vi "ConfigureArmTrigger.vi"(8 "Error In":errorcluster, 10 "Arm Configuration":T1={"Source"=enum."Hold", "Count"=1, "Infinite?"=FALSE} {"Count" min=1 max=99999 step=1}, 11 "Keithley 7001 In":refnum<visa-resource-name>) -> (0 "Error Out":errorcluster, 3 "Keithley 7001 Out":refnum<visa-resource-name>)   [LabVIEW 2012]
uses:
  TriggerArmConfiguration.ctl
  driver/Public/Controls/ArmSource.ctl
  driver/Keithley-7001.lvlib
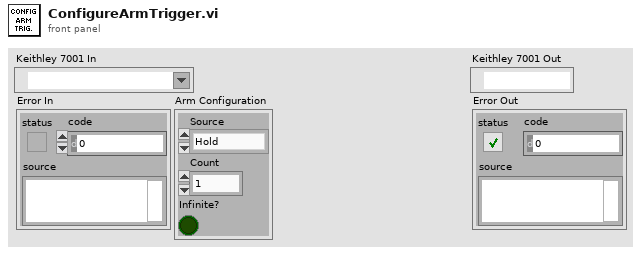
[diagram p1: front panel]
types:
  T1 = typedef "TriggerArmConfiguration.ctl" = cluster{"Source":T2, "Count":u32, "Infinite?":bool}
  T2 = typedef "Keithley-7001.lvlib/ArmSource.ctl" = enum16{"Hold", "Immediate", "Manual", "Bus", "TLink", "External"}
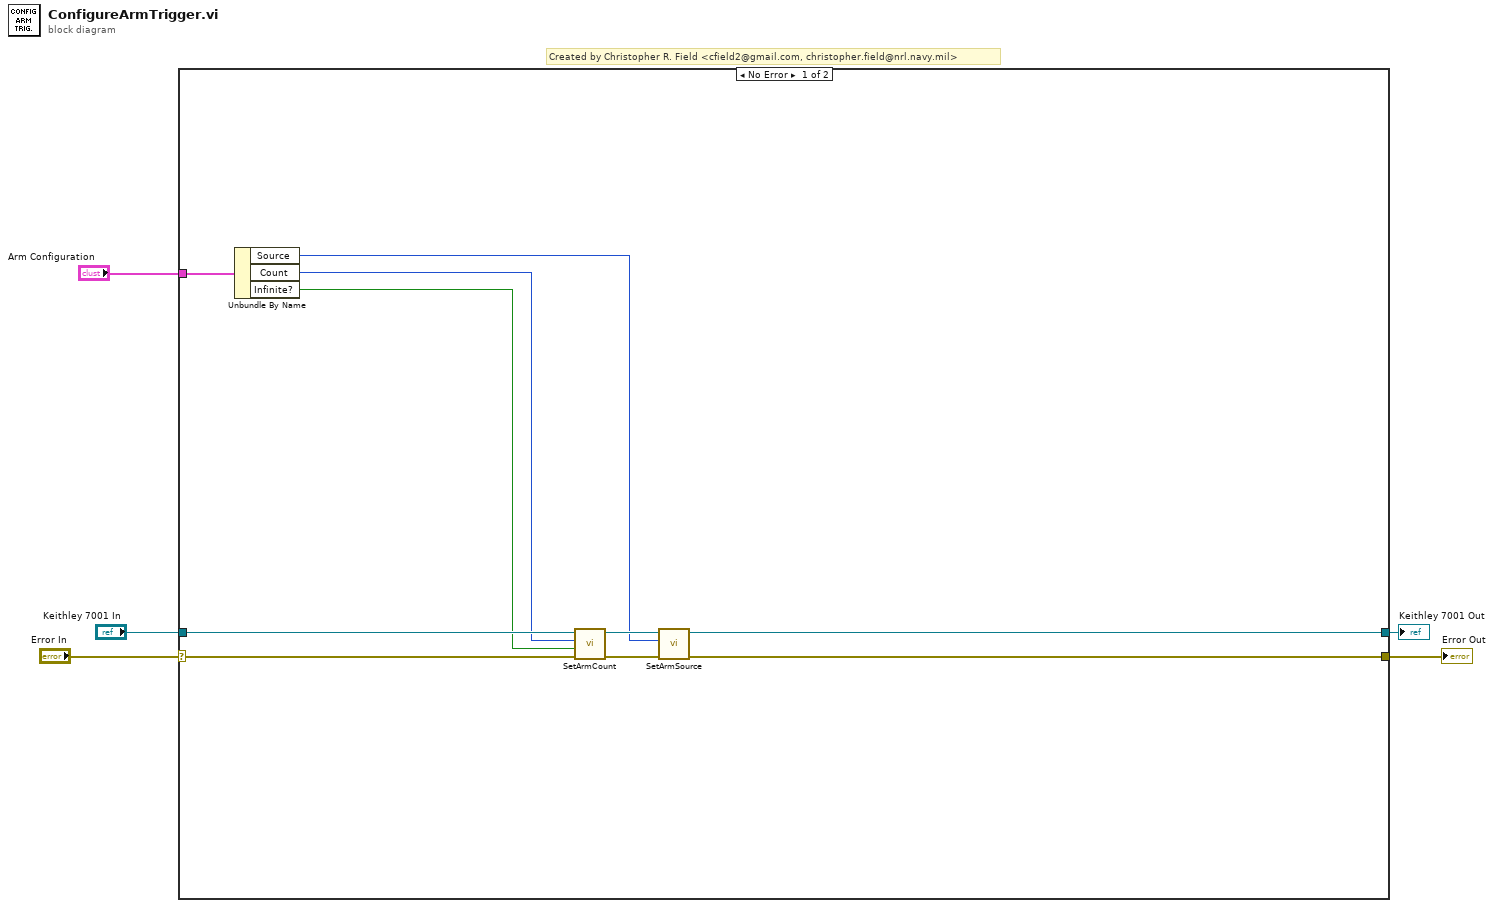
[diagram p0: block diagram]
diagram:
  # "Created by Christopher R. Field <cfield2@gmail.com, christopher.field@nrl.navy.mil>"
  n1 = case shown="No Error" "Error In" {
    selector: "Error In" -> [w12 w16]
    tunnel: "Keithley 7001 In" -> [w13 w17]
    tunnel: [w11 w17] -> w3
    tunnel: [w10 w16] -> w2
    tunnel: "Arm Configuration" -> [w9 _]
    frame No Error {
      n2 = Unbundle By Name(w9) -> ("Source"=w8:T2, "Count"=w7:u32, "Infinite?"=w6:bool)
      n3 = call "SetArmCount.vi"("Error In"=w12, "Infinite?"=w6, "Count (1-9999)"=w7, "Keithley 7001 In"=w13) -> ("Error Out"=w14:errorcluster, "Keithley 7001 Out"=w15:refnum<visa-resource-name>)  [unwired: 6 in]
      n4 = call "SetArmSource.vi"("Error In"=w14, "Source"=w8, "Keithley 7001 In"=w15) -> ("Error Out"=w10:errorcluster, "Keithley 7001 Out"=w11:refnum<visa-resource-name>)  [unwired: 7 in]
    }
    frame Error {
    }
  }
  "Keithley 7001 Out" <- w3
  "Error Out" <- w2
